vi "GetIndexCA.vi"(11 "CA":T1(array[cluster])) -> (2 "N-index":i32, 3 "Current index":u8)   [LabVIEW 2020]
uses:
  Global Variables/Global N-Back Setting.vi
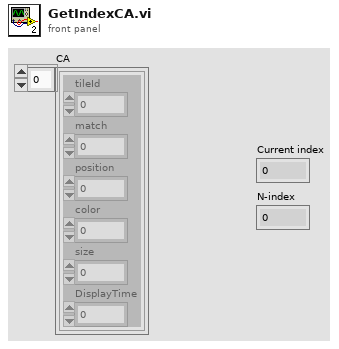
[diagram p1: front panel]
types:
  T1 = cluster{"tileId":i32, "match":i32, "position":i32, "color":u32, "size":i32, "DisplayTime":i32}[]
  T2 = cluster{"tileId":i32, "match":i32, "position":i32, "color":u32, "size":i32, "DisplayTime":i32}
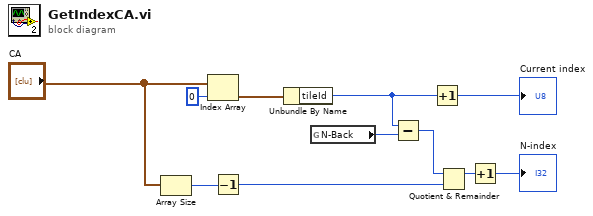
[diagram p0: block diagram]
diagram:
  n1 = Array Size(array="CA") -> (size(s)=w8:i32)
  n2 = Index Array(array="CA", index=0) -> (element=w11:T2)
  n3 = Decrement(x=w8) -> (x-1=w5:i32)
  n4 = Unbundle By Name(w11) -> ("tileId"=w7:i32)
  n5 = global read "Global N-Back Setting.vi" "N-Back"() -> (w2:u8)
  n6 = Subtract(x=w7, y=w2) -> (x-y=w9:i32)
  n7 = Increment(x=w7) -> (x+1=→"Current index":i32)
  n8 = Quotient & Remainder(x=w9, y=w5) -> (x-y*floor(x/y)=w6:i32)  [unwired: 1 out]
  n9 = Increment(x=w6) -> (x+1=→"N-index":i32)
